vi "Sous-vi-Cluster.vi"(3 "Fiche d'identité Write":T1) -> (0 "Fiche d'identité Read":T1, 1 "Sortie_char":string="Sub-VI")   [LabVIEW 2020]
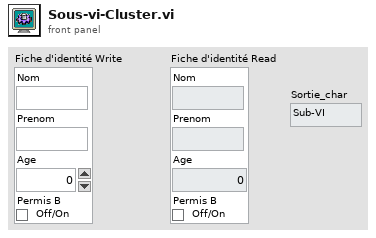
[diagram p1: front panel]
types:
  T1 = cluster{"Nom":string, "Prenom":string, "Age":dbl, "Permis B":bool}
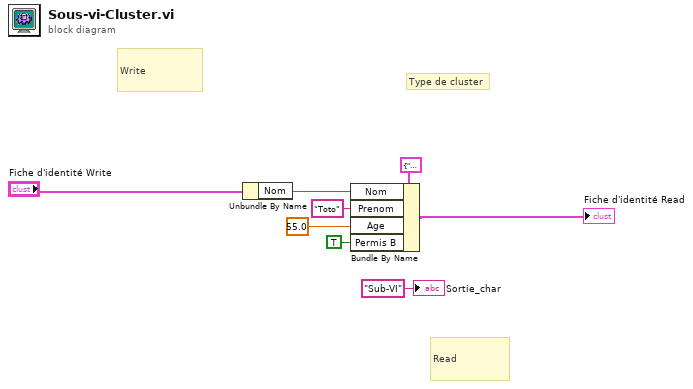
[diagram p0: block diagram]
diagram:
  # "Read"
  # "Write"
  # "Type de cluster"
  n1 = Unbundle By Name("Fiche d'identité Write") -> ("Nom"=w7:string)
  n2 = Bundle By Name(cluster=T1 {"Nom"="0", "Prenom"="0", "Age"=0.0, "Permis B"=FALSE} ("Fiche d'identité Read"), "Nom"=w7, "Prenom"="Toto", "Age"=55.0, "Permis B"=TRUE) -> (→"Fiche d'identité Read":T1)
  "Sortie_char" <- "Sub-VI" ("Prenom")
